vi "New_Group_id_writer.vi"(0 "Enable":bool=TRUE, 1 "Default Group ID":u16(ring) items=["CCLDAS"=1, "LASP"=2, "CU"=3, "NLSI"=4, "LDEX"=5, "Heidelberg"=6], 5 "error in (no error)":errorcluster, 6 "Default Experiment Name":string caption="Please Enter Tags:", 8 "default Experiment Description":string caption="Please Enter Experiment Description:") -> (14 "Cancel 2":bool caption="Cancel", 15 "Please Enter Experiment Description:":string, 16 "Please Enter Tags:":string, 17 "Please Enter Group ID":dbl format="%#g", 18 "OK":bool, 19 "error out":errorcluster)   [LabVIEW 2011]
doc: "Displays a standard dialog box that prompts users to enter information, such as a user name and password.\n--------------------\n\nThis Express VI is configured as follows:\n\nMessage to Display to the User:Please Enter Experiment Settings Information For Database Storage.\nThe inputs are: \nNumber: Please Enter Group ID\nText Entry Box: Please Enter Tags:\nText Entry Box: Please Enter Experiment Description:"
uses:
  <vilib>/addons/database/Connection.llb/Conn Execute.vi
  <vilib>/addons/database/Recordset.llb/Rec Fetch Recordset Data (R).vi
  <vilib>/addons/database/Recordset.llb/Rec Destroy - Connection.vi
  <vilib>/addons/database/_DB Variant To Data/Database Variant To Data.xnode
  <vilib>/addons/database/NI_Database_API.lvlib
panel:
  out "Default Experiment Name 2":string caption="Please Enter Tags:"
  out "default Experiment Description 2":string caption="Please Enter Experiment Description:"
  out "Default Group ID 2":u16(ring) items=["CCLDAS"=1, "LASP"=2, "CU"=3, "NLSI"=4, "LDEX"=5, "Heidelberg"=6]
  in  "Please Select Group:":u16(ring) items=["CCLDAS"=1, "LASP"=2, "CU"=3, "Team Awesome"=4]
  in  "Please Enter an Experiment Description:":string caption="Please Enter Experiment Description:"
  in  "Please Enter an Experiment Name:":string caption="Please Enter Tags:"
  in  "Cancel":bool
  in  "OK2":bool
  in  "OK1":bool
  # "Please Enter Experiment Settings Information For Storage in the CCLDAS Database."
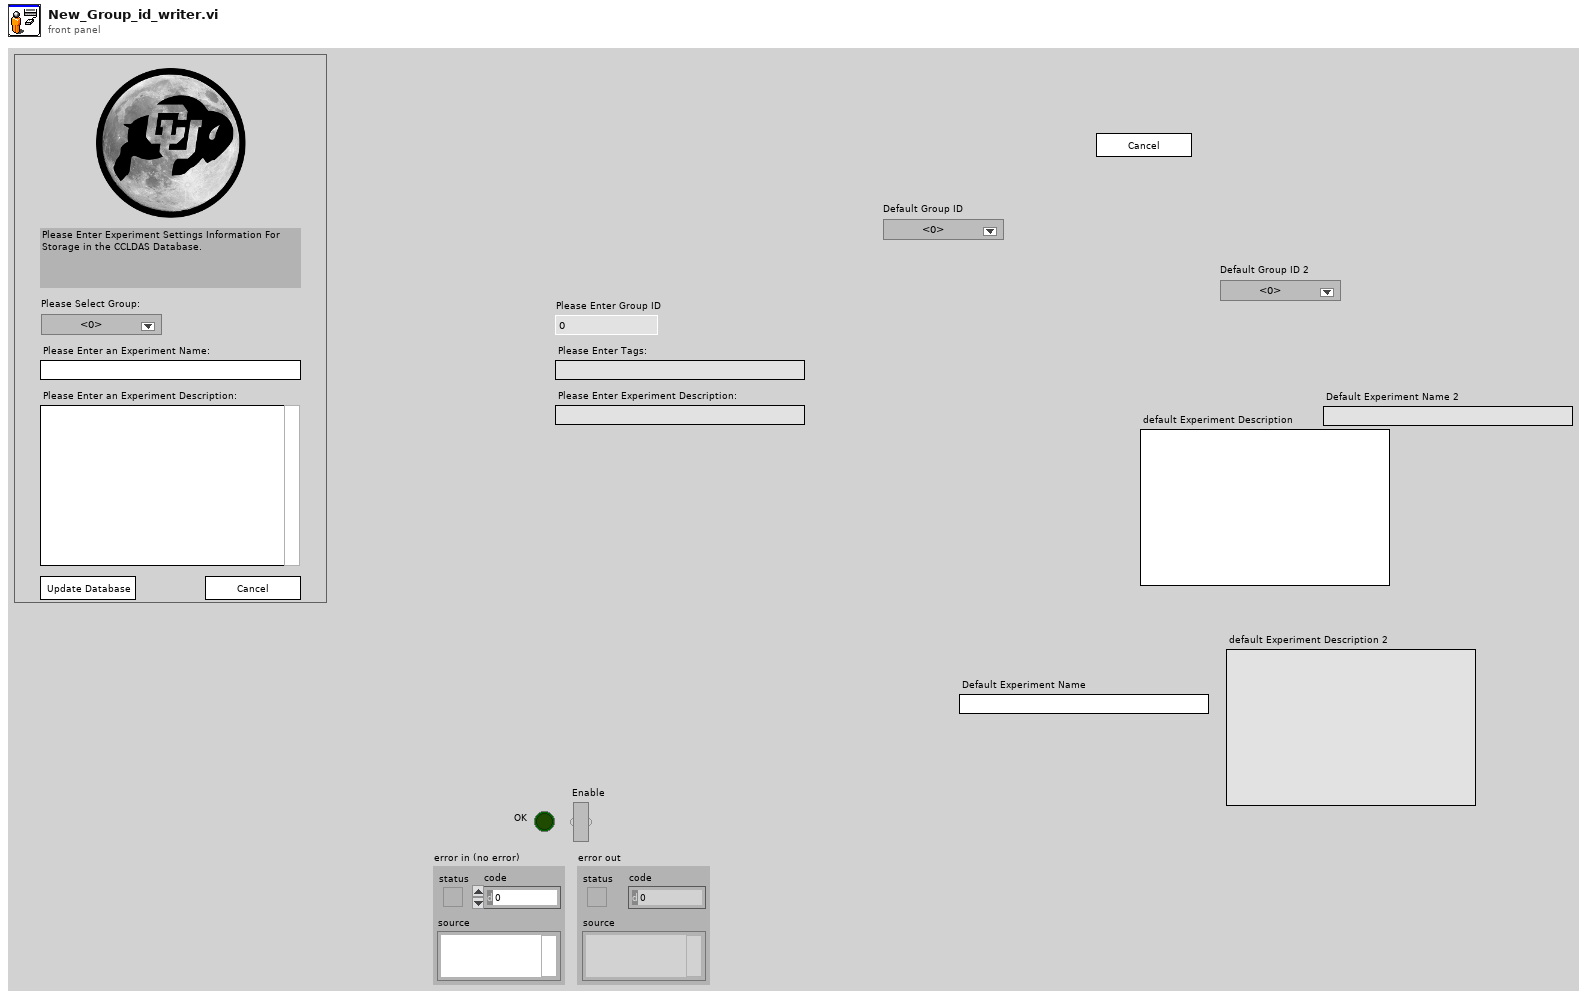
[diagram p1: front panel]
types:
  T1 = typedef "NI_Database_API.lvlib/Conn ObjectReference.ctl" = refnum<k1>
  T2 = typedef "NI_Database_API.lvlib/Rec ObjectReference.ctl" = refnum<k1>
  T3 = cluster{"Input Name":string, "Input Data Type":i32}
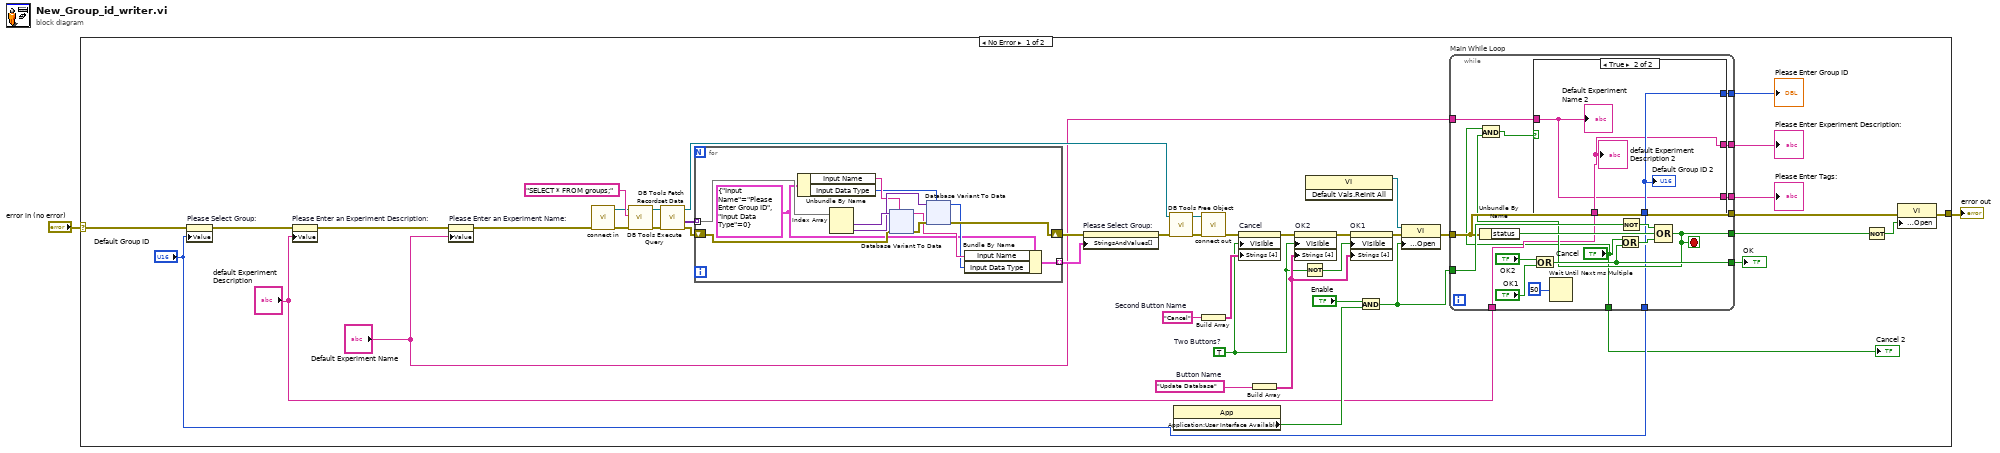
[diagram p0: block diagram]
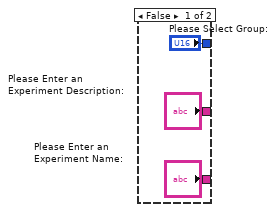
[diagram p2: hidden frame]
diagram:
  n1 = case shown="No Error" "error in (no error)" {
    selector: "error in (no error)" -> [w10 w147]
    tunnel: [w11 w147] -> w1
    frame No Error {
      w20 = "Cancel"  # Second Button Name
      w22 = "Update Database"  # Button Name
      w12 = TRUE  # Two Buttons?
      n2 = property on="Please Select Group:" class="Ring (strict)"(error in=w10, "Value"="Default Group ID") -> (error out=w9:errorcluster)  [unwired: 1 in, 1 out]
      n3 = property on="Please Enter an Experiment Description:" class="Str"(error in=w9, "Value"="default Experiment Description") -> (error out=w8:errorcluster)  [unwired: 1 in, 1 out]
      n4 = property on="Please Enter an Experiment Name:" class="Str"(error in=w8, "Value"="Default Experiment Name") -> (error out=w7:errorcluster)  [unwired: 1 in, 1 out]
      n5 = call "connect in.vi"("error in (no error)"=w7) -> ("error out"=w34:errorcluster, "Database Connection"=w33:T1)  [unwired: 6 in, 1 out]
      n6 = call-poly <vilib>:"DB Tools Execute Query.vi"("error in (no error)"=w34, "SQL query"="SELECT * FROM groups;", "connection reference"=w33) -> ("error out"=w36:errorcluster, "recordset reference"=w35:T2)  [unwired: 5 in]
      n7 = call-poly <vilib>:"DB Tools Fetch Recordset Data.vi"("error in (no error)"=w36, "recordset reference"=w35) -> ("error out"=w43:errorcluster, "recordset data"=w42:variant[][], "recordset reference out"=w37:T2)  [unwired: 3 in]
      n8 = for {
        tunnel: w42 -> [w58] mode=indexing
        shift-right: [w53] -> w44
        shift-left: w43 -> [w54]
        tunnel: [w52] -> w46 mode=indexing
        w47 = T3 {"Input Name"="Please Enter Group ID", "Input Data Type"=0}
        n9 = Unbundle By Name(w47) -> ("Input Name"=w51:string, "Input Data Type"=w48:i32)
        n10 = Index Array(array=w58) -> (element #1=w57:variant, element #2=w56:variant)  [unwired: 2 in]
        n11 = xnode "Database Variant To Data"("database variant"=w57, "error in"=w54, "type"=w51) -> ("data"=w50:string, "error out"=w55:errorcluster)
        n12 = xnode "Database Variant To Data"("database variant"=w56, "error in"=w55, "type"=w48) -> ("data"=w49:i32, "error out"=w53:errorcluster)
        n13 = Bundle By Name(cluster=w47, "Input Name"=w50, "Input Data Type"=w49) -> (w52:T3)
      }
      n14 = property on="Please Select Group:" class="Ring (strict)"(error in=w44, "StringsAndValues[]"=w46) -> (error out=w45:errorcluster)  [unwired: 1 in, 1 out]
      n15 = call-poly <vilib>:"DB Tools Free Object.vi"("error in (no error)"=w45, "recordset reference"=w37) -> ("error out"=w38:errorcluster, "connection reference"=w39:T1)  [unwired: 8 in]
      n16 = property class="App"() -> ("Application:User Interface Available"=w27:bool)  [unwired: 2 in, 2 out]
      n17 = call "connect out.vi"("error in (no error)"=w38, "connection reference"=w39) -> ("error out"=w40:errorcluster)  [unwired: 9 in]
      n18 = Build Array(w20) -> (w19:string[])
      n19 = property on="Cancel" class="Bool"(error in=w40, "Visible"=w12, "Strings [4]"=w19) -> (error out=w15:errorcluster)  [unwired: 1 in, 1 out]
      n20 = Build Array(w22) -> (w21:string[])
      n21 = property on="OK2" class="Bool"(error in=w15, "Visible"=w12, "Strings [4]"=w21) -> (error out=w16:errorcluster)  [unwired: 1 in, 1 out]
      n22 = Not(x=w12) -> (.not. x?=w14:bool)
      n23 = invoke class="VI" method="Default Vals.Reinit All"() -> (reference out=w28:refnum<vi>)  [unwired: 3 in, 2 out]
      n24 = property on="OK1" class="Bool"(error in=w16, "Visible"=w14, "Strings [4]"=w21) -> (error out=w23:errorcluster)  [unwired: 1 in, 1 out]
      n25 = And(x="Enable", y=w27) -> (x .and. y?=w26:bool)
      n26 = property class="VI"(reference=w28, error in=w23, "Front Panel Window:Open"=w26) -> (error out=w32:errorcluster)  [unwired: 1 out]
      n27 = while "Main While Loop" {
        tunnel: [w138] -> w13
        tunnel: w26 -> [w136]
        tunnel: [w127] -> w18
        tunnel: w32 -> [w134]
        tunnel: [w134] -> w24
        tunnel: [w129] -> w29
        tunnel: [w131] -> w30
        tunnel: [w130] -> w31
        tunnel: "Default Experiment Name" -> [w126]
        tunnel: "default Experiment Description" -> [w125]
        tunnel: "Default Group ID" -> [w124]
        tunnel: ["Cancel"] -> w3
        stop <- w127 stop-if-true
        n28 = Unbundle By Name(w134) -> ("status"=w132:bool)
        n29 = Or(x="OK2", y="OK1") -> (x .or. y?=w138:bool)
        n30 = Wait Until Next ms Multiple(millisecond multiple=u32 50) -> ()  [unwired: 1 out]
        n31 = Or(x="Cancel", y=w138) -> (x .or. y?=w133:bool)
        n32 = Not(x=w136) -> (.not. x?=w135:bool)
        n33 = Compound Arithmetic op=OR(w135, w132, w133) -> (w127:bool)
        n34 = And(x="Cancel", y=w127) -> (x .and. y?=w128:bool)
        n35 = case shown="True" w128 {
          tunnel: ["Please Enter an Experiment Name:" w144] -> w131
          tunnel: ["Please Enter an Experiment Description:" w145] -> w130
          tunnel: ["Please Select Group:" w146] -> w129
          tunnel: w126 -> [_ w144]
          tunnel: w125 -> [_ w145]
          tunnel: w124 -> [_ w146]
          frame False {
          }
          frame True {
            "Default Group ID 2" <- w146
            "default Experiment Description 2" <- w145
            "Default Experiment Name 2" <- w144
          }
        }
      }
      "OK" <- w13
      "Please Enter Group ID" <- w29
      "Please Enter Tags:" <- w30
      "Please Enter Experiment Description:" <- w31
      "Cancel 2" <- w3
      n36 = Not(x=w18) -> (.not. x?=w17:bool)
      n37 = property class="VI"(error in=w24, "Front Panel Window:Open"=w17) -> (error out=w11:errorcluster)  [unwired: 1 in, 1 out]
    }
    frame Error {
    }
  }
  "error out" <- w1
